vi "CMD CfgDaq.vi"(8 "error in (no error)":errorcluster, 9 "AI TaskName":string, 10 "AI InstSettings":T1, 11 "DAQ in":refnum<class "DAQ.lvclass">) -> (0 "error out":errorcluster, 3 "DAQ out":refnum<class "DAQ.lvclass">)   [LabVIEW 2017, in "DAQ.lvclass"]
doc: "Developed by Kevin Thompson\nkevin@thompsonengineering.net\n\nCopyright 2018-2020\nThompson Engineering, LLC"
uses:
  DAQ.lvclass
  DataTypes/TD AI InstSettings--cluster.ctl
  DataTypes/AsyncCmd_DAQ--enum.ctl
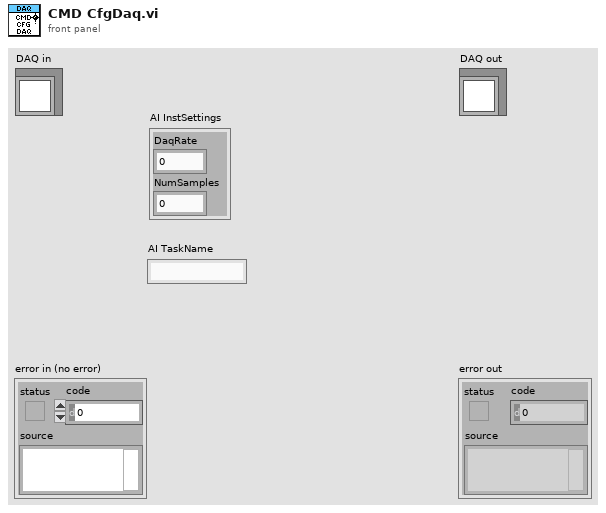
[diagram p1: front panel]
types:
  T1 = typedef "DAQ.lvclass/TD AI InstSettings--cluster.ctl" = cluster{"DaqRate":dbl, "NumSamples":i32}
  T2 = typedef "DAQ.lvclass/AsyncCmd_DAQ--enum.ctl" = enum16{"StartDAQ", "StopDAQ", "CfgDAQ"}
  T3 = cluster{"AI InstSettings":T1, "AI TaskName":string}
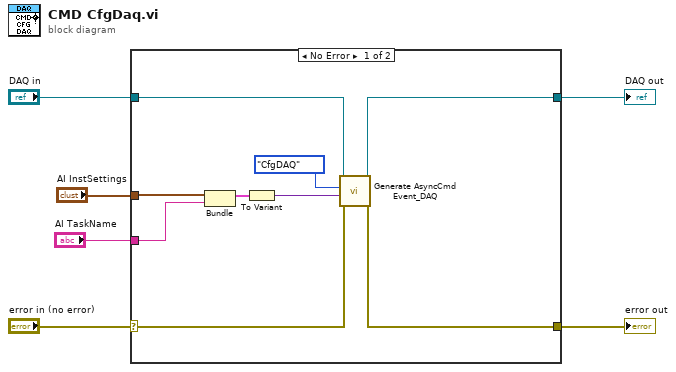
[diagram p0: block diagram]
diagram:
  n1 = case shown="No Error" "error in (no error)" {
    selector: "error in (no error)" -> [w15 w17]
    tunnel: [w14 w17] -> w5
    tunnel: [w12 w16] -> w3
    tunnel: "DAQ in" -> [w13 w16]
    tunnel: "AI InstSettings" -> [w8 _]
    tunnel: "AI TaskName" -> [w7 _]
    frame No Error {
      n2 = Bundle("AI InstSettings"=w8, "AI TaskName"=w7) -> (w9:T3)  [unwired: 1 in]
      n3 = To Variant(anything=w9) -> (Variant=w10:variant)
      n4 = call "Generate AsyncCmd Event_DAQ.vi"("error in (no error)"=w15, "vData"=w10, "AsyncCmd"=AsyncCmd_DAQ--enum."CfgDAQ" ("AsyncMsg"), "DAQ"=w13) -> ("error out"=w14:errorcluster, "DAQ out"=w12:refnum<class "DAQ.lvclass">)  [unwired: 6 in]
    }
    frame Error {
    }
  }
  "error out" <- w5
  "DAQ out" <- w3
